vi "Drop Element.vi"(8 "error in (no error)":errorcluster, 10 "Drop Element":T1, 11 "Test Executive Builder Model in":refnum<class "Test Executive Builder Model.lvclass">) -> (0 "error out":errorcluster, 3 "Test Executive Builder Model out":refnum<class "Test Executive Builder Model.lvclass">, 5 "Unique ID":string)   [LabVIEW 2019, in "Test Executive Builder Model.lvclass"]
uses:
  <vilib>/gpm_packages/@cs/Test-executive-builder/Source/Test Executive Builder Model/Test Executive Builder Model/Test Executive Builder Model.lvclass
  C:/Program Files/National Instruments/LabVIEW 2019/vi.lib/ActorFramework/Actor/Actor.lvclass
  <vilib>/gpm_packages/@cs/Test-executive-builder/Source/Application Dependencies/Drop Element.ctl
  <vilib>/gpm_packages/@cs/Test-executive-builder/Source/Test Executive Builder Model/Test Executive Builder Model/Test Executive Builder Model.lvclass/Test Executive Builder Model.ctl
  <vilib>/ActorFramework/Actor/Actor.lvclass/Actor.ctl
  <vilib>/ActorFramework/Message Enqueuer/Message Enqueuer.lvclass/Message Enqueuer.ctl
  <vilib>/ActorFramework/Message Enqueuer/Init from Existing Queue.vi
  <vilib>/ActorFramework/Message Enqueuer/Enqueue.vi
  <vilib>/gpm_packages/@cs/Test-executive-builder/Source/Test Executive Builder Model/Test Executive Builder Model Messages/Redraw Tree Msg/Redraw Tree Msg.lvclass
  C:/Program Files/National Instruments/LabVIEW 2019/vi.lib/ActorFramework/Message/Message.lvclass
  <vilib>/ActorFramework/Message Priority Queue/Priority Enqueue.vi
  <vilib>/ActorFramework/Message Enqueuer/Message Enqueuer.lvclass
  <vilib>/gpm_packages/@cs/test-executive/Source/Test Executive/TestExecutive Ref/TestExecutive Ref.lvclass
  <vilib>/ActorFramework/Actor/Actor.lvclass
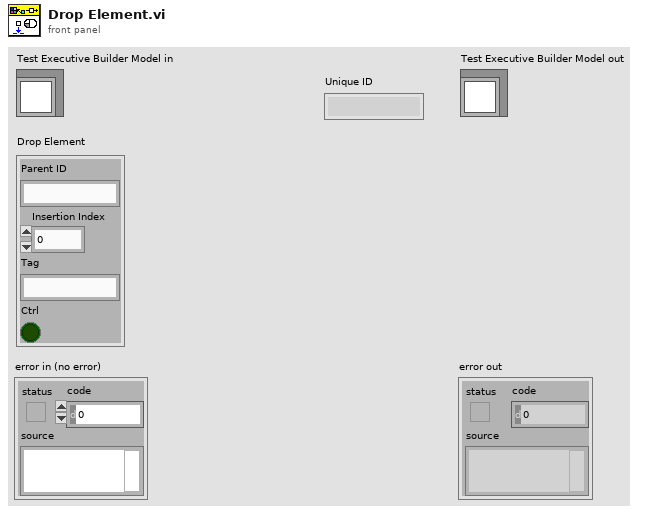
[diagram p1: front panel]
types:
  T1 = typedef "Drop Element.ctl" = cluster{"Parent ID":string, "Insertion Index":i32, "Tag":string, "Ctrl":bool}
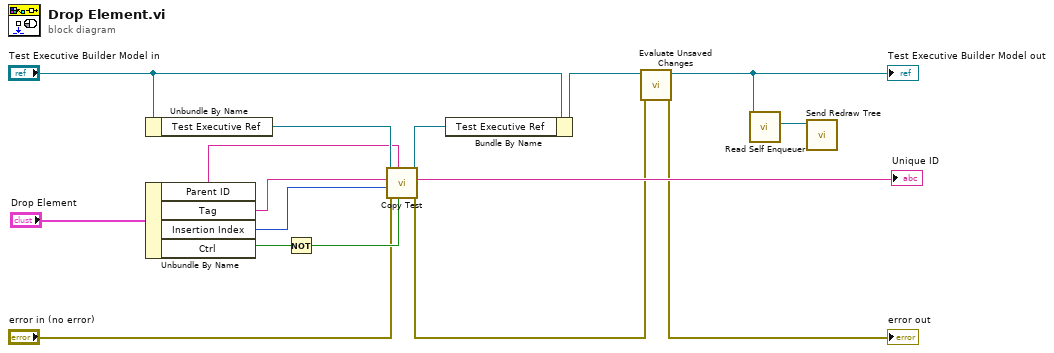
[diagram p0: block diagram]
diagram:
  n1 = Unbundle By Name("Test Executive Builder Model in") -> ("Test Executive Ref"=w16:refnum<data-value>)
  n2 = Unbundle By Name("Drop Element") -> ("Parent ID"=w14:string, "Tag"=w13:string, "Insertion Index"=w12:i32, "Ctrl"=w11:bool)
  n3 = Not(x=w11) -> (.not. x?=w10:bool)
  n4 = call <vilib>:"Copy Test.vi"("Move?"=w10, "New Parent ID"=w14, "error in (no error)"="error in (no error)", "Insertion Index"=w12, "Test ID"=w13, "Test Executive Ref"=w16) -> ("error out"=w2:errorcluster, "Test ID out"=→"Unique ID":string, "Test Executive Ref out"=w15:refnum<data-value>)  [unwired: 3 in]
  n5 = Bundle By Name(cluster="Test Executive Builder Model in", "Test Executive Ref"=w15) -> (w4:refnum<class "Test Executive Builder Model.lvclass">)
  n6 = call-dynamic "Evaluate Unsaved Changes.vi"("error in (no error)"=w2, "Test Executive Builder Model in"=w4) -> ("error out"=→"error out":errorcluster, "Test Executive Builder Model out"=w3:refnum<class "Test Executive Builder Model.lvclass">)  [unwired: 8 in]
  "Test Executive Builder Model out" <- w3
  n7 = call <vilib>:"Read Self Enqueuer.vi"("Actor"=w3) -> ("Self Enqueuer"=w9:refnum<class "Message Enqueuer.lvclass">)  [unwired: 10 in]
  n8 = call <vilib>:"Send Redraw Tree.vi"("Message Enqueuer"=w9) -> ()  [unwired: 9 in, 2 out]
